vi "roi_feedback.vi"(1 "output cluster":T1) -> (0 "destination":i16[][](array[numeric]))   [LabVIEW 2015]
uses:
  MWT.dll
panel:
  out "return type 2":i32
  out "return type":i32
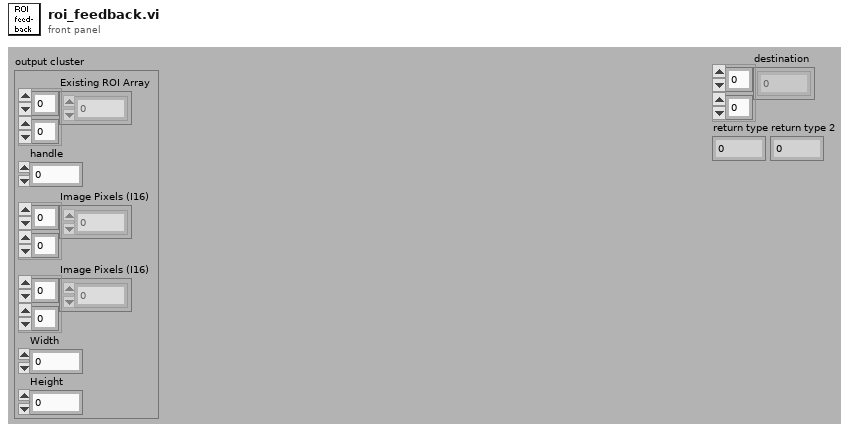
[diagram p1: front panel]
types:
  T1 = cluster{"Existing ROI Array":dbl[][], "handle":i32, "Image Pixels (I16)":i16[][], "Image Pixels (I16)":i16[][], "Width":u32, "Height":u32}
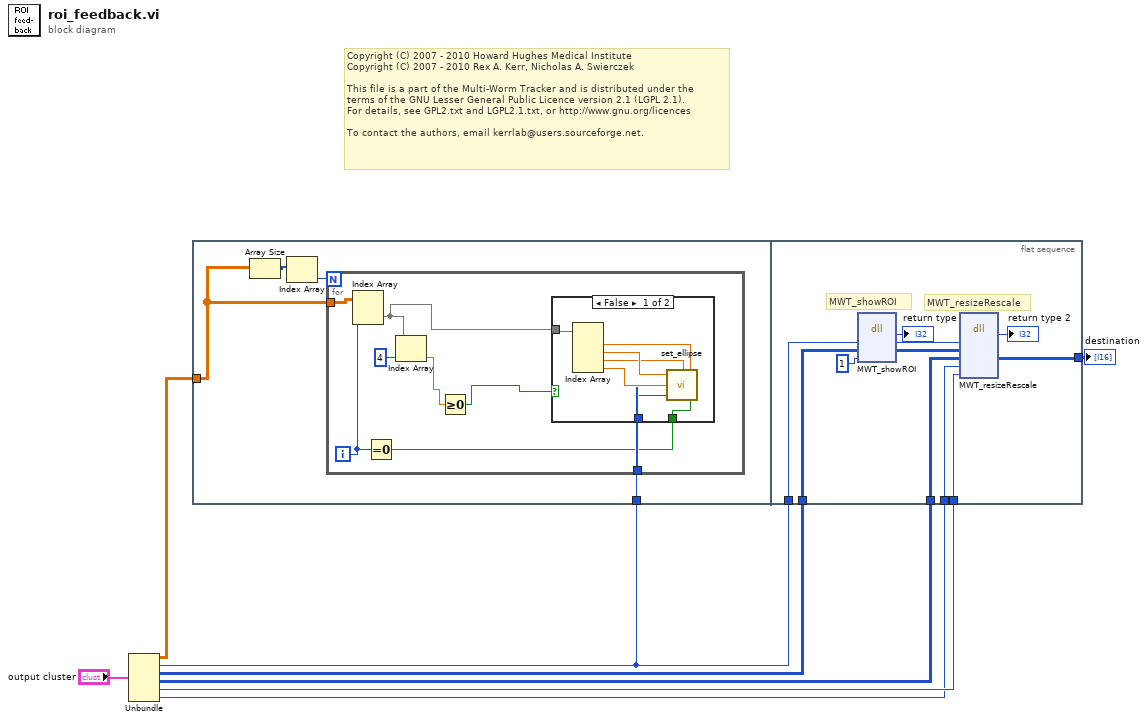
[diagram p0: block diagram]
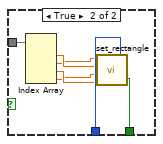
[diagram p2: hidden frame]
diagram:
  # "Copyright (C) 2007 - 2010 Howard Hughes Medical Institute\nCopyright (C) 2007 - 2010 Rex A. Kerr, Nicholas A. Swierczek\n \nThis file is a part of the Multi-Worm Tracker and is distributed under the\nterms of the GNU Lesser General Public Licence version 2.1 (LGPL 2.1).\nFor details, see GPL2.txt and LGPL2.1.txt, or http://www.gnu.org/licences\n \nTo contact the authors, email kerrlab@users.sourceforge.net."
  n1 = Unbundle("output cluster") -> ("Existing ROI Array"=w8:dbl[][], "handle"=w5:i32, "Image Pixels (I16)"=w7:i16[][], "Image Pixels (I16)"=w6:i16[][], "Width"=w2:u32, "Height"=w1:u32)
  n2 = flat-sequence {
    tunnel: w5 -> [w12]
    tunnel: w8 -> [w11]
    tunnel: [w43] -> w4
    tunnel: w5 -> [w42]
    tunnel: w7 -> [w40]
    tunnel: w6 -> [w39]
    tunnel: w1 -> [w38]
    tunnel: w2 -> [w37]
    frame #0 {
      n3 = Array Size(array=w11) -> (size(s)=w10:i32[])
      n4 = Index Array(array=w10) -> (element=w9:i32)  [unwired: 1 in]
      n5 = for {
        N: w9 -> [_]
        tunnel: w11 -> [w18]
        tunnel: w12 -> [w20]
        i -> [w16]
        n6 = Index Array(array=w18, index (row)=w16) -> (element=w17:dbl[])  [unwired: 1 in]
        n7 = Equal To 0?(x=w16) -> (x = 0?=w19:bool)
        n8 = Index Array(array=w17, index=4) -> (element=w13:dbl)
        n9 = Greater Or Equal To 0?(x=w13) -> (x >= 0?=w15:bool)
        n10 = case shown="False" w15 {
          tunnel: w17 -> [w27 w34]
          tunnel: w20 -> [w22 w33]
          tunnel: w19 -> [w21 w32]
          frame False {
            n11 = Index Array(array=w27) -> (element #1=w26:dbl, element #2=w25:dbl, element #3=w24:dbl, element #4=w23:dbl)  [unwired: 4 in]
            n12 = call "set_ellipse.vi"("Set/Add"=w21, "y2"=w24, "y1"=w26, "Handle"=w22, "x2"=w23, "x1"=w25) -> ()
          }
          frame True {
            n13 = Index Array(array=w34) -> (element #1=w31:dbl, element #2=w30:dbl, element #3=w29:dbl, element #4=w28:dbl)  [unwired: 4 in]
            n14 = call "set_rectangle.vi"("Set/Add"=w32, "Handle"=w33, "y2"=w29, "x2"=w28, "y1"=w31, "x1"=w30) -> ()
          }
        }
      }
    }
    frame #1 {
      # "MWT_resizeRescale"
      # "MWT_showROI"
      n15 = dll-call lib="C:/_WORKSPACE/DATA/PROJECTS/IMAQ/SOFTWARE/MWT NO STIM/MWT.dll" fn="MWT_showROI"("handle"=w42, "image"=w40, "bin"=1) -> ("return type"=→"return type":i32, "handle"=w44:i32, "image"=w45:i16[][])  [unwired: 4 in, 2 out]
      n16 = dll-call lib="C:/_WORKSPACE/DATA/PROJECTS/IMAQ/SOFTWARE/MWT NO STIM/MWT.dll" fn="MWT_resizeRescale"("handle"=w44, "source"=w45, "destination"=w39, "width"=w38, "height"=w37) -> ("return type"=→"return type 2":i32, "destination"=w43:i16[][])  [unwired: 7 in, 2 out]
    }
  }
  "destination" <- w4
